vi "KE622x -- Set Service Request Event Enable Reg State.vi"(0 "VISA Resource In":refnum<visa-resource-name>, 1 "Error Query (T)?":bool=TRUE, 7 "KE622x Service Request Enable Reg State":T1, 11 "error in (no error)":errorcluster) -> (4 "VISA Resource Out (dupl)":refnum<visa-resource-name>, 15 "error out":errorcluster)   [LabVIEW 2019, in "Keithley 622x.lvlib"]
doc: "Sets the bits in the 'Service Request Enable' register of the Status Model. Note that only the used (named) bits are settable -- all other bits default to zero."
uses:
  Keithley 622x.lvlib
  Typedefs/KE622x -- Service Request Enable Reg State.ctl
panel:
  out "Reg Num (dec)":u8 format="%0d"
  out "Reg Num (binary)":u8 format="%016b"
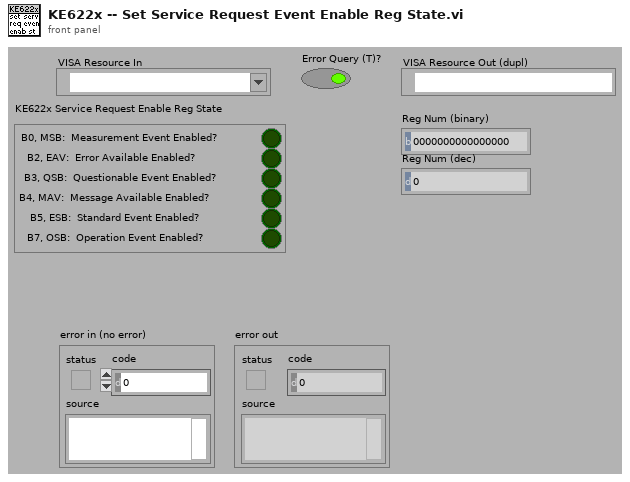
[diagram p1: front panel]
types:
  T1 = typedef "Keithley 622x.lvlib/KE622x -- Service Request Enable Reg State.ctl" = cluster{"B0, MSB:  Measurement Event Enabled?":bool, "B2, EAV:  Error Available Enabled?":bool, "B3, QSB:  Questionable Event Enabled?":bool, "B4, MAV:  Message Available Enabled?":bool, "B5, ESB:  Standard Event Enabled?":bool, "B7, OSB:  Operation Event Enabled?":bool}
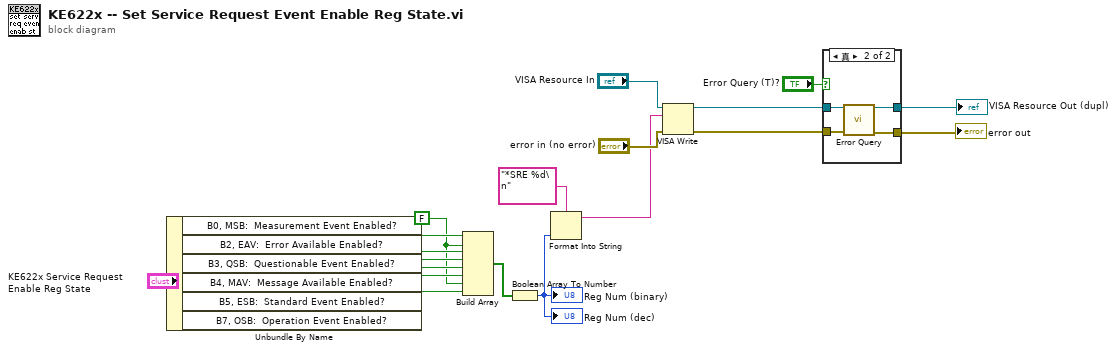
[diagram p0: block diagram]
diagram:
  w6 = FALSE
  n1 = Unbundle By Name("KE622x Service Request Enable Reg State") -> ("B0, MSB:  Measurement Event Enabled?"=w12:bool, "B2, EAV:  Error Available Enabled?"=w11:bool, "B3, QSB:  Questionable Event Enabled?"=w10:bool, "B4, MAV:  Message Available Enabled?"=w9:bool, "B5, ESB:  Standard Event Enabled?"=w8:bool, "B7, OSB:  Operation Event Enabled?"=w7:bool)
  n2 = Build Array(w12, w6, w11, w10, w9, w8, w6, w7) -> (w18:bool[])
  n3 = Boolean Array To Number(Boolean array=w18) -> (number=w15:u32)
  "Reg Num (binary)" <- w15
  "Reg Num (dec)" <- w15
  n4 = Format Into String(format string="*SRE %d\n" ("write buffer"), w15) -> (resulting string=w13:string)  [unwired: 2 in, 1 out]
  n5 = VISA Write(VISA resource name="VISA Resource In", write buffer=w13, error in (no error)="error in (no error)") -> (VISA resource name out=w4:refnum<visa-resource-name>, error out=w3:errorcluster)  [unwired: 1 out]
  n6 = case shown="真" "Error Query (T)?" {
    tunnel: w3 -> [w20 w25]
    tunnel: w4 -> [w21 w24]
    tunnel: [w20 w23] -> w1
    tunnel: [w21 w22] -> w2
    frame False {
    }
    frame True {
      n7 = call "Error Query.vi"("VISA Resource In"=w24, "error in (no error)"=w25) -> ("VISA Resource Out (dupl)"=w22:refnum<visa-resource-name>, "error out"=w23:errorcluster)  [unwired: 10 in, 2 out]
    }
  }
  "VISA Resource Out (dupl)" <- w2
  "error out" <- w1
